vi "BRig_dataTrial_Cue2_n.vi"() -> (2 "output_Cue2_n":i32)   [LabVIEW 2014]
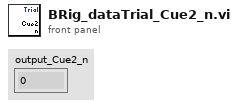
[diagram p1: front panel]
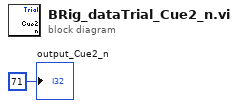
[diagram p0: block diagram]
diagram:
  "output_Cue2_n" <- 71 ("output_iBlock")
